vi "Part 1.vi"(11 "Input":string) -> (3 "Output":i64)   [LabVIEW 2021]
uses:
  <userlib>/_OpenG.lib/array/array.llb/Search 1D Array (String)__ogtk.vi
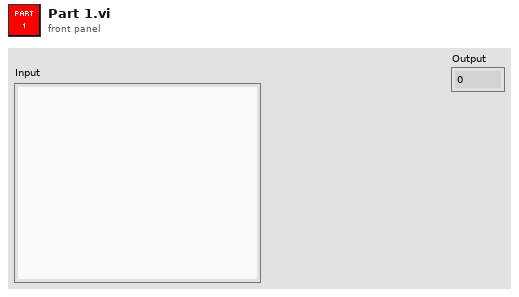
[diagram p1: front panel]
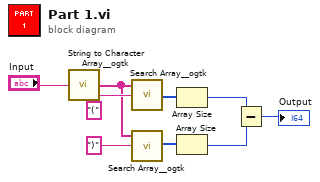
[diagram p0: block diagram]
diagram:
  n1 = call <userlib>:"String to Character Array__ogtk.vi"("Input String"="Input") -> ("Character Array"=w6:string[])
  n2 = call-poly <userlib>:"Search Array__ogtk.vi"("Array"=w6, "Element Data"="(") -> ("Indices of Elements"=w5:i32[])  [unwired: 7 in]
  n3 = call-poly <userlib>:"Search Array__ogtk.vi"("Array"=w6, "Element Data"=")") -> ("Indices of Elements"=w4:i32[])  [unwired: 7 in]
  n4 = Array Size(array=w5) -> (size(s)=w3:i32)
  n5 = Array Size(array=w4) -> (size(s)=w2:i32)
  n6 = Subtract(x=w3, y=w2) -> (x-y=→"Output":i32)
